vi "Key Down - Delete Row.vi"(8 "error in (no error)":errorcluster, 9 "Action Keys (Delete)":T1[](array[typedef])=[enum."Delete"], 10 "Key Pressed in":T1, 11 "MCListbox with Checkboxes in":refnum<class "MCListbox with Checkboxes.lvclass">) -> (0 "error out":errorcluster, 2 "Key Pressed out":T1, 3 "MCListbox with Checkboxes out":refnum<class "MCListbox with Checkboxes.lvclass">)   [LabVIEW 2016, in "MCListbox with Checkboxes.lvclass"]
uses:
  MCListbox with Checkboxes.lvclass
  <vilib>/event_ctls.llb/eventvkey.ctl
  MCListbox with Checkboxes.lvclass/MCListbox with Checkboxes.ctl
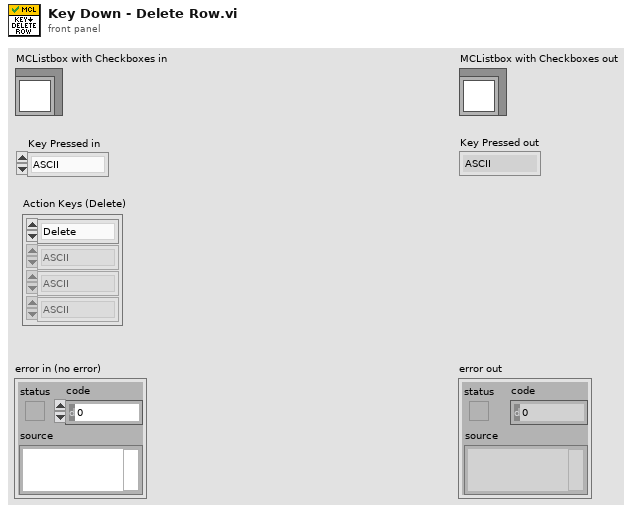
[diagram p1: front panel]
types:
  T1 = typedef "eventvkey.ctl" = enum16{"ASCII", "Enter", "Return", "Shift", "Ctrl", "Alt", "Cmd", "Opt", "Caps", "NumLock", "Clear", "Break", "Up", "Down", "Left", "Right", "Insert", "Delete", "Home", "End", "PageUp", "PageDown", "Escape", "Help", "Pause", "ScrollLock", "F1", "F2", "F3", "F4", "F5", "F6", "F7", "F8", "F9", "F10", "F11", "F12", "F13", "F14", "F15", "F16", "F17", "F18", "F19", "F20", "F21", "F22", "F23", "F24", "Play", "VolumeUp", "VolumeDown", "Mute", "Two Byte Char"}
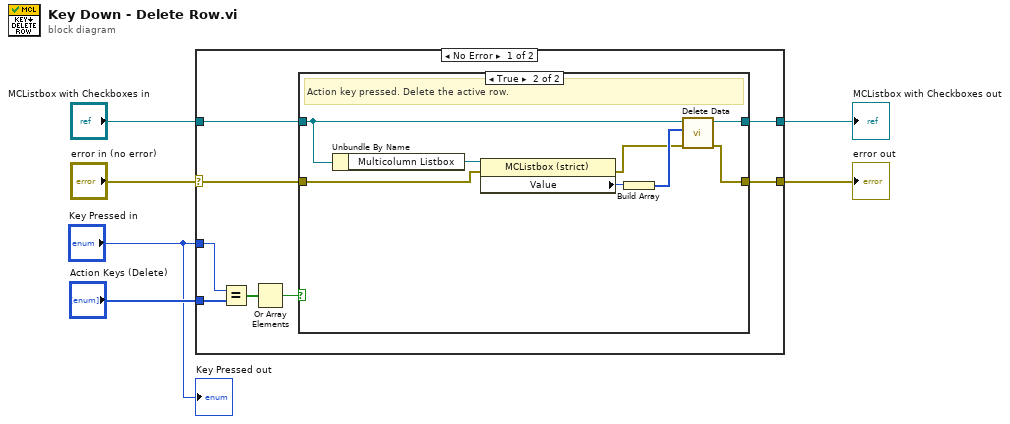
[diagram p0: block diagram]
diagram:
  n1 = case shown="No Error" "error in (no error)" {
    selector: "error in (no error)" -> [w8 w26]
    tunnel: [w7 w26] -> w5
    tunnel: [w9 w25] -> w3
    tunnel: "MCListbox with Checkboxes in" -> [w10 w25]
    tunnel: "Action Keys (Delete)" -> [w13 _]
    tunnel: "Key Pressed in" -> [w14 _]
    frame No Error {
      n2 = Equal?(x=w14, y=w13) -> (x = y?=w12:bool[])
      n3 = Or Array Elements(Boolean array=w12) -> (logical OR=w11:bool)
      n4 = case shown="True" w11 {
        tunnel: w10 -> [w16 w22]
        tunnel: [w16 w20] -> w9
        tunnel: w8 -> [w15 w19]
        tunnel: [w15 w17] -> w7
        frame False {
          # "Action key not pressed. Do nothing."
        }
        frame True {
          # "Action key pressed. Delete the active row."
          n5 = Unbundle By Name(w22) -> ("Multicolumn Listbox"=w23:refnum<vi>)
          n6 = property class="MCListbox (strict)"(reference=w23, error in=w19) -> (error out=w18:errorcluster, "Value"=w24:i32)  [unwired: 1 out]
          n7 = Build Array(w24) -> (w21:i32[])
          n8 = call "Delete Data.vi"("error in (no error)"=w18, "Rows"=w21, "MCListbox with Checkboxes in"=w22) -> ("error out"=w17:errorcluster, "MCListbox with Checkboxes out"=w20:refnum<class "MCListbox with Checkboxes.lvclass">)  [unwired: 7 in]
        }
      }
    }
    frame Error {
    }
  }
  "error out" <- w5
  "MCListbox with Checkboxes out" <- w3
  "Key Pressed out" <- "Key Pressed in"
